vi "FindSpacing.vi"(11 "All Code":string) -> (1 "indent?":bool, 2 "spaces":i32, 3 "length of cmd":i32)   [LabVIEW 2019]
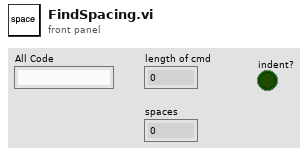
[diagram p1: front panel]
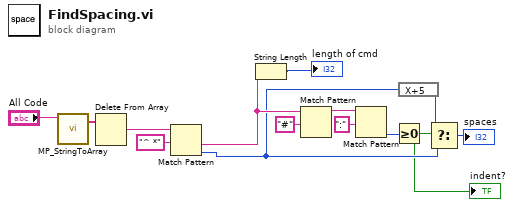
[diagram p0: block diagram]
diagram:
  n1 = call <userlib>:"MP_StringToArray.vi"("write buffer"="All Code") -> ("Array"=w1:string[])  [unwired: 10 in]
  n2 = Delete From Array(array=w1) -> (deleted portion=w3:string)  [unwired: 2 in, 1 out]
  n3 = Match Pattern(string=w3, regular expression="^ *") -> (after substring=w12:string, offset past match=w11:i32)  [unwired: 1 in, 2 out]
  n4 = String Length(string=w12) -> (length=→"length of cmd":i32)
  n5 = Match Pattern(string=w12, regular expression="#") -> (before substring=w10:string)  [unwired: 1 in, 3 out]
  n6 = Match Pattern(string=w10, regular expression=":") -> (offset past match=w6:i32)  [unwired: 1 in, 3 out]
  n7 = Greater Or Equal To 0?(x=w6) -> (x >= 0?=w7:bool)
  "indent?" <- w7
  n8 = expression code="X+5"(w11) -> (w8:i32)
  n9 = Select(t=w8, s=w7, f=w11) -> (s? t:f=→"spaces":i32)
